vi "SetConfig.vi"(8 "error in (no error)":errorcluster, 10 "Config":variant, 11 "FitterBase in":refnum<class "FitterBase.lvclass">) -> (0 "error out":errorcluster, 3 "FitterBase out":refnum<class "FitterBase.lvclass">)   [LabVIEW 2018, in "AnalysisPlugins.lvlib" / "FitterBase.lvclass"]
uses:
  FitterBase.lvclass
  Y:/Projects/PMUCal/Modules/Analysis/AnalysisPlugins/AnalysisPluginBaseClass/AnalysisPluginsBase.lvclass
  Typedefs/clAnalysisConfig.ctl
  AnalysisPluginBaseClass/AnalysisPluginsBase.lvclass/AnalysisPluginsBase.ctl
  AnalysisPluginBaseClass/Accessors/Read AnalysisConfig.vi
  AnalysisPluginBaseClass/Accessors/Write AnalysisConfig.vi
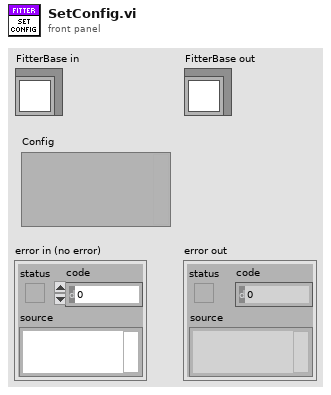
[diagram p1: front panel]
types:
  T1 = typedef "AnalysisPlugins.lvlib/FitterBase.lvclass/clAnalysisConfig.ctl" = cluster{"F0":u32, "SettlingTime":dbl, "AnalysisCycles":dbl, "SampleRate":dbl, "NumChannels":u32, "TsOffset":enum16{"start", "middle", "end"}}
  T2 = cluster{"F0":u32, "SettlingTime":dbl, "AnalysisCycles":dbl, "SampleRate":dbl, "NumChannels":u32}
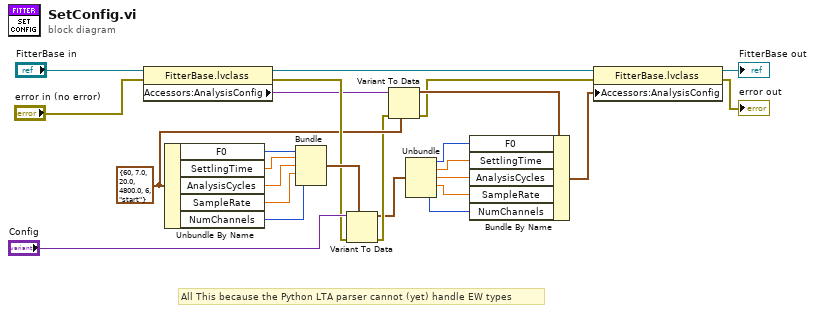
[diagram p0: block diagram]
diagram:
  w15 = T1 {"F0"=60, "SettlingTime"=7.0, "AnalysisCycles"=20.0, "SampleRate"=4800.0, "NumChannels"=6, "TsOffset"=enum."start"} ("clAnalysisConfig")
  # "All This because the Python LTA parser cannot (yet) handle EW types"
  n1 = property class="FitterBase.lvclass"(reference="FitterBase in", error in="error in (no error)") -> (reference out=w5:refnum<class "FitterBase.lvclass">, error out=w16:errorcluster, "Accessors:AnalysisConfig"=w14:variant)
  n2 = Unbundle By Name(w15) -> ("F0"=w23:u32, "SettlingTime"=w22:dbl, "AnalysisCycles"=w21:dbl, "SampleRate"=w20:dbl, "NumChannels"=w19:u32)
  n3 = Bundle("F0"=w23, "SettlingTime"=w22, "AnalysisCycles"=w21, "SampleRate"=w20, "NumChannels"=w19) -> (w18:T2)  [unwired: 1 in]
  n4 = Variant To Data(error in=w16, type=w18, Variant="Config") -> (data=w12:T2, error out=w13:errorcluster)
  n5 = Variant To Data(error in=w13, type=w15, Variant=w14) -> (data=w11:T1, error out=w1:errorcluster)
  n6 = Unbundle(w12) -> ("F0"=w10:u32, "SettlingTime"=w9:dbl, "AnalysisCycles"=w8:dbl, "SampleRate"=w7:dbl, "NumChannels"=w6:u32)
  n7 = Bundle By Name(cluster=w11, "F0"=w10, "SettlingTime"=w9, "AnalysisCycles"=w8, "SampleRate"=w7, "NumChannels"=w6) -> (w2:T1)
  n8 = property class="FitterBase.lvclass"(reference=w5, error in=w1, "Accessors:AnalysisConfig"=w2) -> (reference out=→"FitterBase out":refnum<class "FitterBase.lvclass">, error out=→"error out":errorcluster)
